vi "PixelsToRealWorldCoordinates.vi"(7 "error in (no error)":errorcluster, 9 "Pixels":dbl[][](array[numeric]), 10 "Calibration 2":T1={"Pixel Width (X)"=1.0, "Pixel Height (Y)"=1.0}) -> (0 "error out":errorcluster, 3 "Real World Points":dbl[][](array[numeric]))   [LabVIEW 2017, in "ImageAcquisitionLibrary.lvlib"]
uses:
  ImageAcquisitionLibrary.lvlib
  Settings/Calibration.ctl
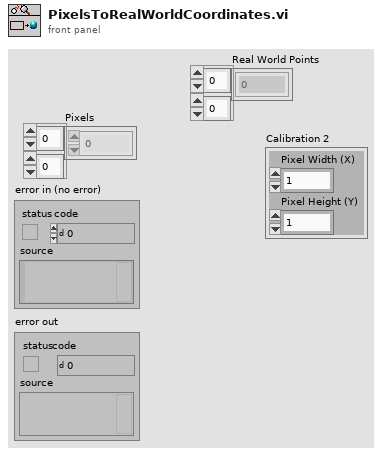
[diagram p1: front panel]
types:
  T1 = typedef "ImageAcquisitionLibrary.lvlib/Calibration.ctl" = cluster{"Pixel Width (X)":dbl, "Pixel Height (Y)":dbl}
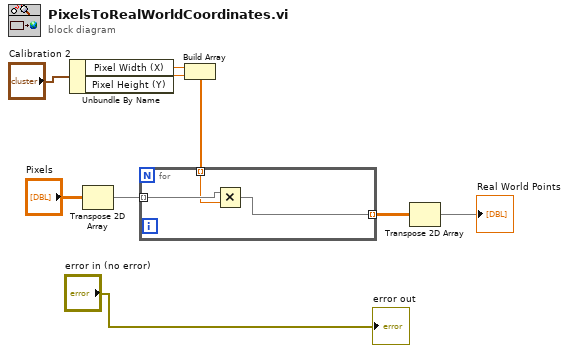
[diagram p0: block diagram]
diagram:
  n1 = Unbundle By Name("Calibration 2") -> ("Pixel Width (X)"=w9:dbl, "Pixel Height (Y)"=w8:dbl)
  n2 = Transpose 2D Array(2D array="Pixels") -> (transposed array=w4:dbl[][])
  n3 = Build Array(w9, w8) -> (w7:dbl[])
  n4 = for {
    tunnel: [w10] -> w3 mode=indexing
    tunnel: w4 -> [w12] mode=indexing
    tunnel: w7 -> [w11] mode=indexing
    n5 = Multiply(x=w12, y=w11) -> (x*y=w10:dbl[])
  }
  n6 = Transpose 2D Array(2D array=w3) -> (transposed array=→"Real World Points":dbl[][])
  "error out" <- "error in (no error)"
